vi "CMN_toBufmgr.vi"(0 "command":string, 1 "bufname":string, 5 "arg":string, 7 "bufpointer":u64, 9 "bufsize":u64, 11 "error in":errorcluster, 12 "responseQ":string, 13 "ms timeout (-1)":i32=-1) -> (6 "buffer":T1, 8 "resp error":errorcluster, 15 "error out":errorcluster)   [LabVIEW 2016]
panel:
  in  "response struct":T2
  in  "commandStruct":T3
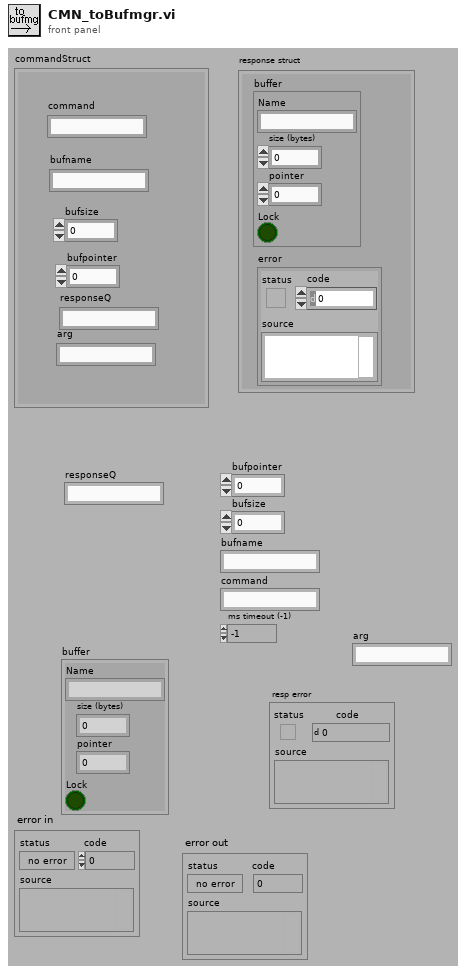
[diagram p1: front panel]
types:
  T1 = cluster{"Name":string, "size (bytes)":u64, "pointer":u64, "Lock":bool}
  T2 = cluster{"buffer":cluster{"Name":string, "size (bytes)":u64, "pointer":u64, "Lock":bool}, "error ":errorcluster}
  T3 = cluster{"command":string, "bufname":string, "bufsize":u64, "bufpointer":u64, "responseQ":string, "arg":string}
  T4 = cluster{"Name":string, "size (bytes)":u32, "pointer":u32, "Lock":bool}
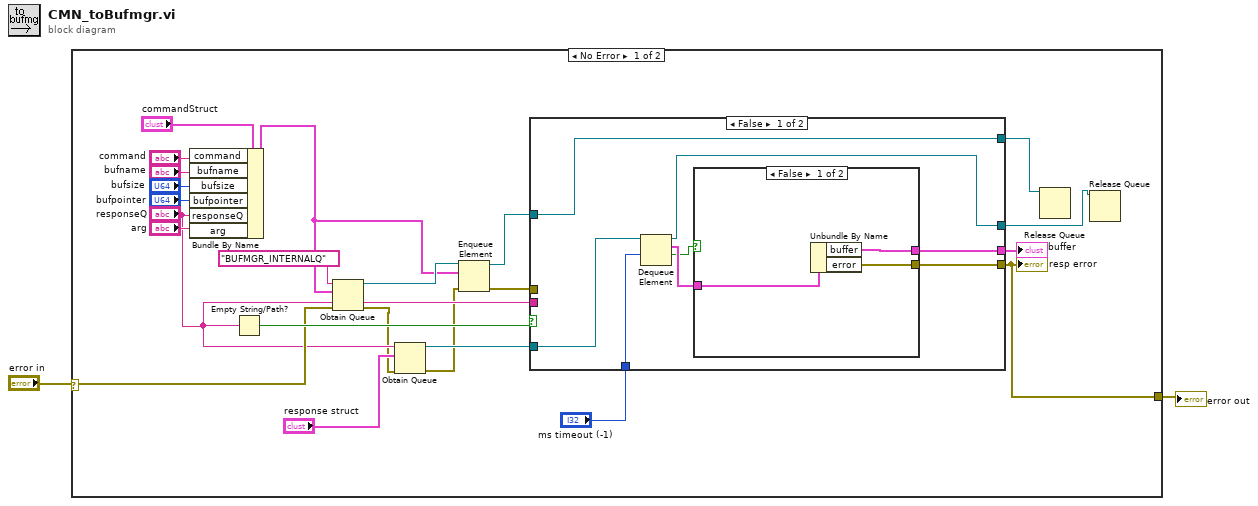
[diagram p0: block diagram]
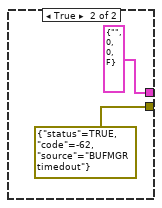
[diagram p2: hidden frame]
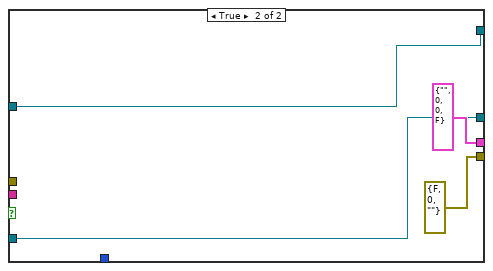
[diagram p3: hidden frame]
diagram:
  n1 = case shown="No Error" "error in" {
    selector: "error in" -> [w14 w43]
    tunnel: [w16 w43] -> w1
    frame No Error {
      n2 = Bundle By Name(cluster="commandStruct", "command"="command", "bufname"="bufname", "bufsize"="bufsize", "bufpointer"="bufpointer", "responseQ"="responseQ", "arg"="arg") -> (w11:T3)
      n3 = Empty String/Path?(string/path="responseQ") -> (empty?=w20:bool)
      n4 = Obtain Queue(name (unnamed)="BUFMGR_INTERNALQ", element data type=w11, error in (no error)=w14) -> (queue out=w12:refnum<queue>, error out=w5:errorcluster)  [unwired: 2 in, 1 out]
      n5 = Obtain Queue(name (unnamed)="responseQ", element data type="response struct", error in (no error)=w5) -> (queue out=w6:refnum<queue>, error out=w4:errorcluster)  [unwired: 2 in, 1 out]
      n6 = Enqueue Element(queue=w12, element=w11, error in (no error)=w4) -> (queue out=w10:refnum<queue>, error out=w13:errorcluster)  [unwired: 2 out]
      n7 = case shown="False" w20 {
        tunnel: "responseQ" -> [_ _]
        tunnel: "ms timeout (-1)" -> [w31 _]
        tunnel: [w33 T1 {"Name"="", "size (bytes)"=0, "pointer"=0, "Lock"=FALSE} ("buffer")] -> w18
        tunnel: [w32 errorcluster {"status"=FALSE, "code"=0, "source"=""} ("error")] -> w16
        tunnel: w13 -> [_ _]
        tunnel: w10 -> [w28 w40]
        tunnel: [w28 w40] -> w9
        tunnel: w6 -> [w27 w39]
        tunnel: [w26 w39] -> w3
        frame False {
          n8 = Dequeue Element(queue=w27, timeout in ms (-1)=w31) -> (queue out=w26:refnum<queue>, element=w30:T2, timed out?=w29:bool)  [unwired: 1 in, 1 out]
          n9 = case shown="False" w29 {
            tunnel: [w36 T4 {"Name"="", "size (bytes)"=0, "pointer"=0, "Lock"=FALSE} ("buffer")] -> w33
            tunnel: [w35 errorcluster {"status"=TRUE, "code"=-62, "source"="BUFMGR timedout"} ("error")] -> w32
            tunnel: w30 -> [w34 _]
            frame False {
              n10 = Unbundle By Name(w34) -> ("buffer"=w36:T1, "error"=w35:errorcluster)
            }
            frame True {
            }
          }
        }
        frame True {
        }
      }
      "buffer" <- w18
      "resp error" <- w16
      n11 = Release Queue(queue=w9) -> ()  [unwired: 1 in, 4 out]
      n12 = Release Queue(queue=w3) -> ()  [unwired: 1 in, 4 out]
    }
    frame Error {
    }
  }
  "error out" <- w1
